vi "Saccade suppression - continuous flash.vi"() -> ()   [LabVIEW 2013]
uses:
  <vilib>/Platform/TimedLoop/XDataNode/timing_clust.ctl
  <vilib>/Platform/TimedLoop/XDataNode/nitl_modes.ctl
  <vilib>/Platform/TimedLoop/XDataNode/wakeup.ctl
  <vilib>/gmath/statdist.llb/Uniform (Discrete) Random.vi
  Eye tracking dependencies/Global 1.vi
  <vilib>/platform/TimedLoop/XDataNode/XDataNode.xnode
  <vilib>/Platform/TimedLoop/XDataNode/XDNodeRunTimeDep.lvlib
  <vilib>/gmath/NI_Gmath.lvlib
panel:
  out "Eye tracker":bool=TRUE
  out "Std name":string="70915_animal15-21_exp1"
  out "Blank":bool
  out "Total number of trials":i32=200
  out "Running!":bool
  in  "Location":string="D:\\Satoru\\Documents\\Attention_Beh_Data\\"
  out "File name exists!":bool
  out "Current trial #":u16
  out "LED":bool
  in  "Abort":bool caption="run-stop"
  in  "File name":string="animal15-29_exp1"
  in  "Save data":bool
  out "State Missed":bool
  out "VS missed":bool
  out "State busy":bool
  out "VS busy":bool
  in  "Tab Control":T1(tab)=enum."Network"
  in  "Notes":string
  in  "Start recording @":string
  in  "Inserted probe @":string
  in  "Brain region":string
  in  "Anesthesia @":string
  in  "Anesthesia":string
  in  "Probe configuration":string
  in  "Probe use number":string
  in  "Probe ID":string
  in  "Probe type":string
  in  "Electrode spacing":string
  in  "Electrode area":string
  in  "Penetration angle (to pia)":string
  in  "Penetration coordinates":string
  in  "Penetration distance":string
  in  "Penetration number":string
  in  "Genotype":string
  in  "Transfection":string
  in  "Mass":string
  in  "Sex":string
  in  "Age":string
  in  "Animal ID":string="14-4"
  in  "inter flash interval (ms)":dbl=300.0
  in  "Max jitter (ms)":dbl=250.0
  in  "VS type":string="continuous_flash"
  in  "Background luminance":sgl
  in  "Pulse amp 0":sgl
  in  "Pulse amp 1":sgl
  in  "Pulse delay (ms)":sgl
  in  "Pulse width (ms)":sgl
  in  "Pulse period":sgl
  in  "Pulse #":sgl
  in  "LED mode":u16(ring) items=["No LED", "Regular", "Random"]
  in  "Chance (%)":dbl
  in  "# of trials":i32=200
  in  "run-stop":bool
  in  "movement":sgl=3.0
  in  "Flash luminance":sgl=100.0
  in  "flash duration (ms)":dbl=48.0
  in  "VS subtype":string="fullfield"
  in  "Include blanks":bool=TRUE
  in  "# of blank trials":i32=200
  in  "Give reward":bool
  in  "Manually give shock":bool
  in  "Water duration (ms)":u32=30
  in  "Shock duration (ms)":u32=10
  in  "Water refractory period (ms)":u32=500
  in  "Shock refractory period (ms)":u32=1000
  in  "Trial timeout (ms)":u32=3000
  in  "Track eye":bool=TRUE
  in  "Allow shock":bool
  in  "Allow timeout":bool
  in  "Manually give water":bool
  in  "Reward period (ms)":u32
  in  "Reward start delay (ms)":u32
  in  "Lick threshold (V)":fxp<+,32,16>=1.600006103515625
  in  "VS threshold (V)":fxp<+,32,16>=0.5
  out "Originating IP":string="192.168.137.2"
  out "Incoming data":string="TrlDone 1.000 "
  in  "Update cycle (ms)":dbl=50.0
  in  "Local IP_This computer":string="192.168.137.10"
  in  "Remote IP_Broadcast":string="192.168.137.255"
  in  "Remote IP_State machine":string="192.168.137.2"
  in  "Remote IP_Visual stimulation":string="192.168.137.3"
  in  "Local port":u16=9090
  in  "Remote port":u16=9091
  out "Error 2":string
  # "Saccade suppression project"
  # "Current trial"
  # "of"
  # "System Status"
  # "VS"
  # "State machine"
  # "Busy"
  # "Missed trial"
  # "Max 20 characters"
  # "(w/o LED)"
  # "Movement threshold (degrees)"
  # "MAX 199.9988"
  # "(This will add trials to the # of trials specified above)"
  # "Errors for debugging"
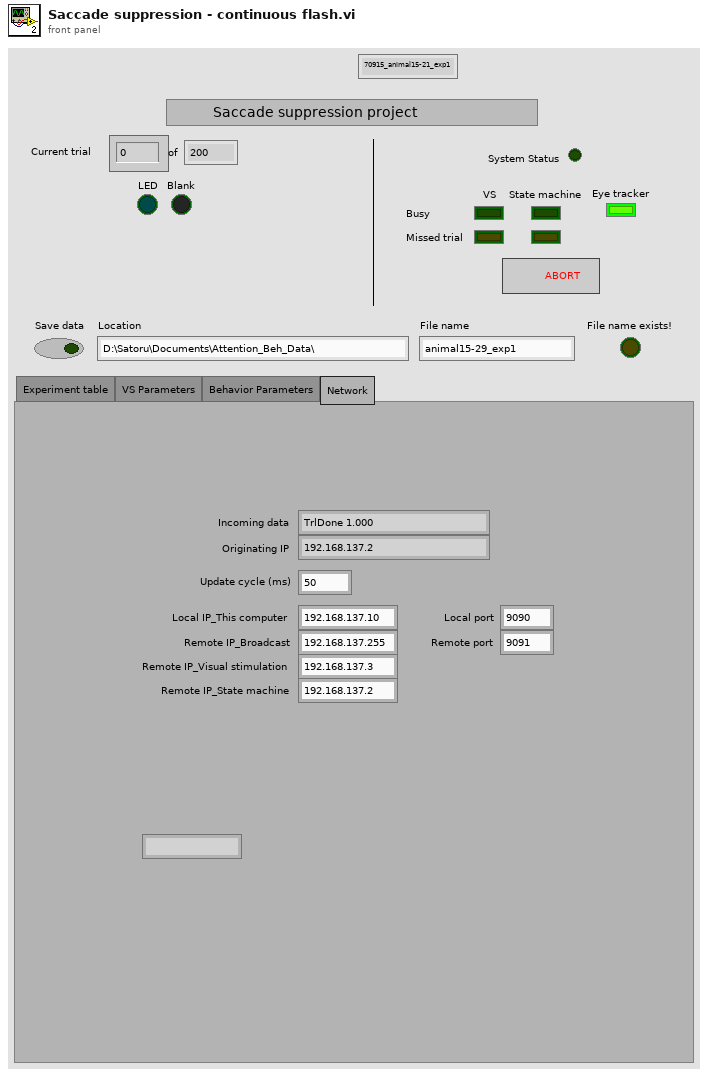
[diagram p1: front panel]
types:
  T1 = enum32{"Experiment table", "VS Parameters", "Behavior Parameters", "Network"}
  T2 = typedef "XDNodeRunTimeDep.lvlib/timing_clust.ctl" = cluster{"Expected End [f-1]":u64, "Actual End [f-1]":u64, "Finished Late? [f-1]":bool, "Expected End [i-1]":u64, "Actual End [i-1]":u64, "Finished Late? [i-1]":bool, "Expected Start [i]":u64, "Actual Start [i]":u64, "Expected Start [f]":u64, "Actual Start [f]":u64, "Source Name":string, "Structure Name":string, "Period":i64, "Deadline":i64, "Offset":i64, "Start":i64, "Priority":i32, "Timeout":i32, "Mode":T3, "Wakeup Reason":T4, "Error":errorcluster, "Source Type":string, "Secondary Source Type":string, "Global End Time":u64, "Global Start Time":u64, "Frame Duration":u64, "Iteration Duration":u64, "Assigned CPU":i32, "I/O Scan Engine Mode":u32}
  T3 = typedef "XDNodeRunTimeDep.lvlib/nitl_modes.ctl" = enum32{"No Change", "Process missed periods, maintain original phase", "Discard missed periods, maintain original phase", "Process missed periods, ignore original phase", "Discard missed periods, ignore original phase"}
  T4 = typedef "XDNodeRunTimeDep.lvlib/wakeup.ctl" = enum32{"Normal", "Aborted", "Asynchronous wakeup", "Timing source error", "Timed loop error", "Timeout"}
  T5 = enum16{"big-endian, network order", "native, host order", "little-endian"}
  T6 = enum16{"open", "replace", "create", "open or create", "replace or create", "replace or create with confirmation"}
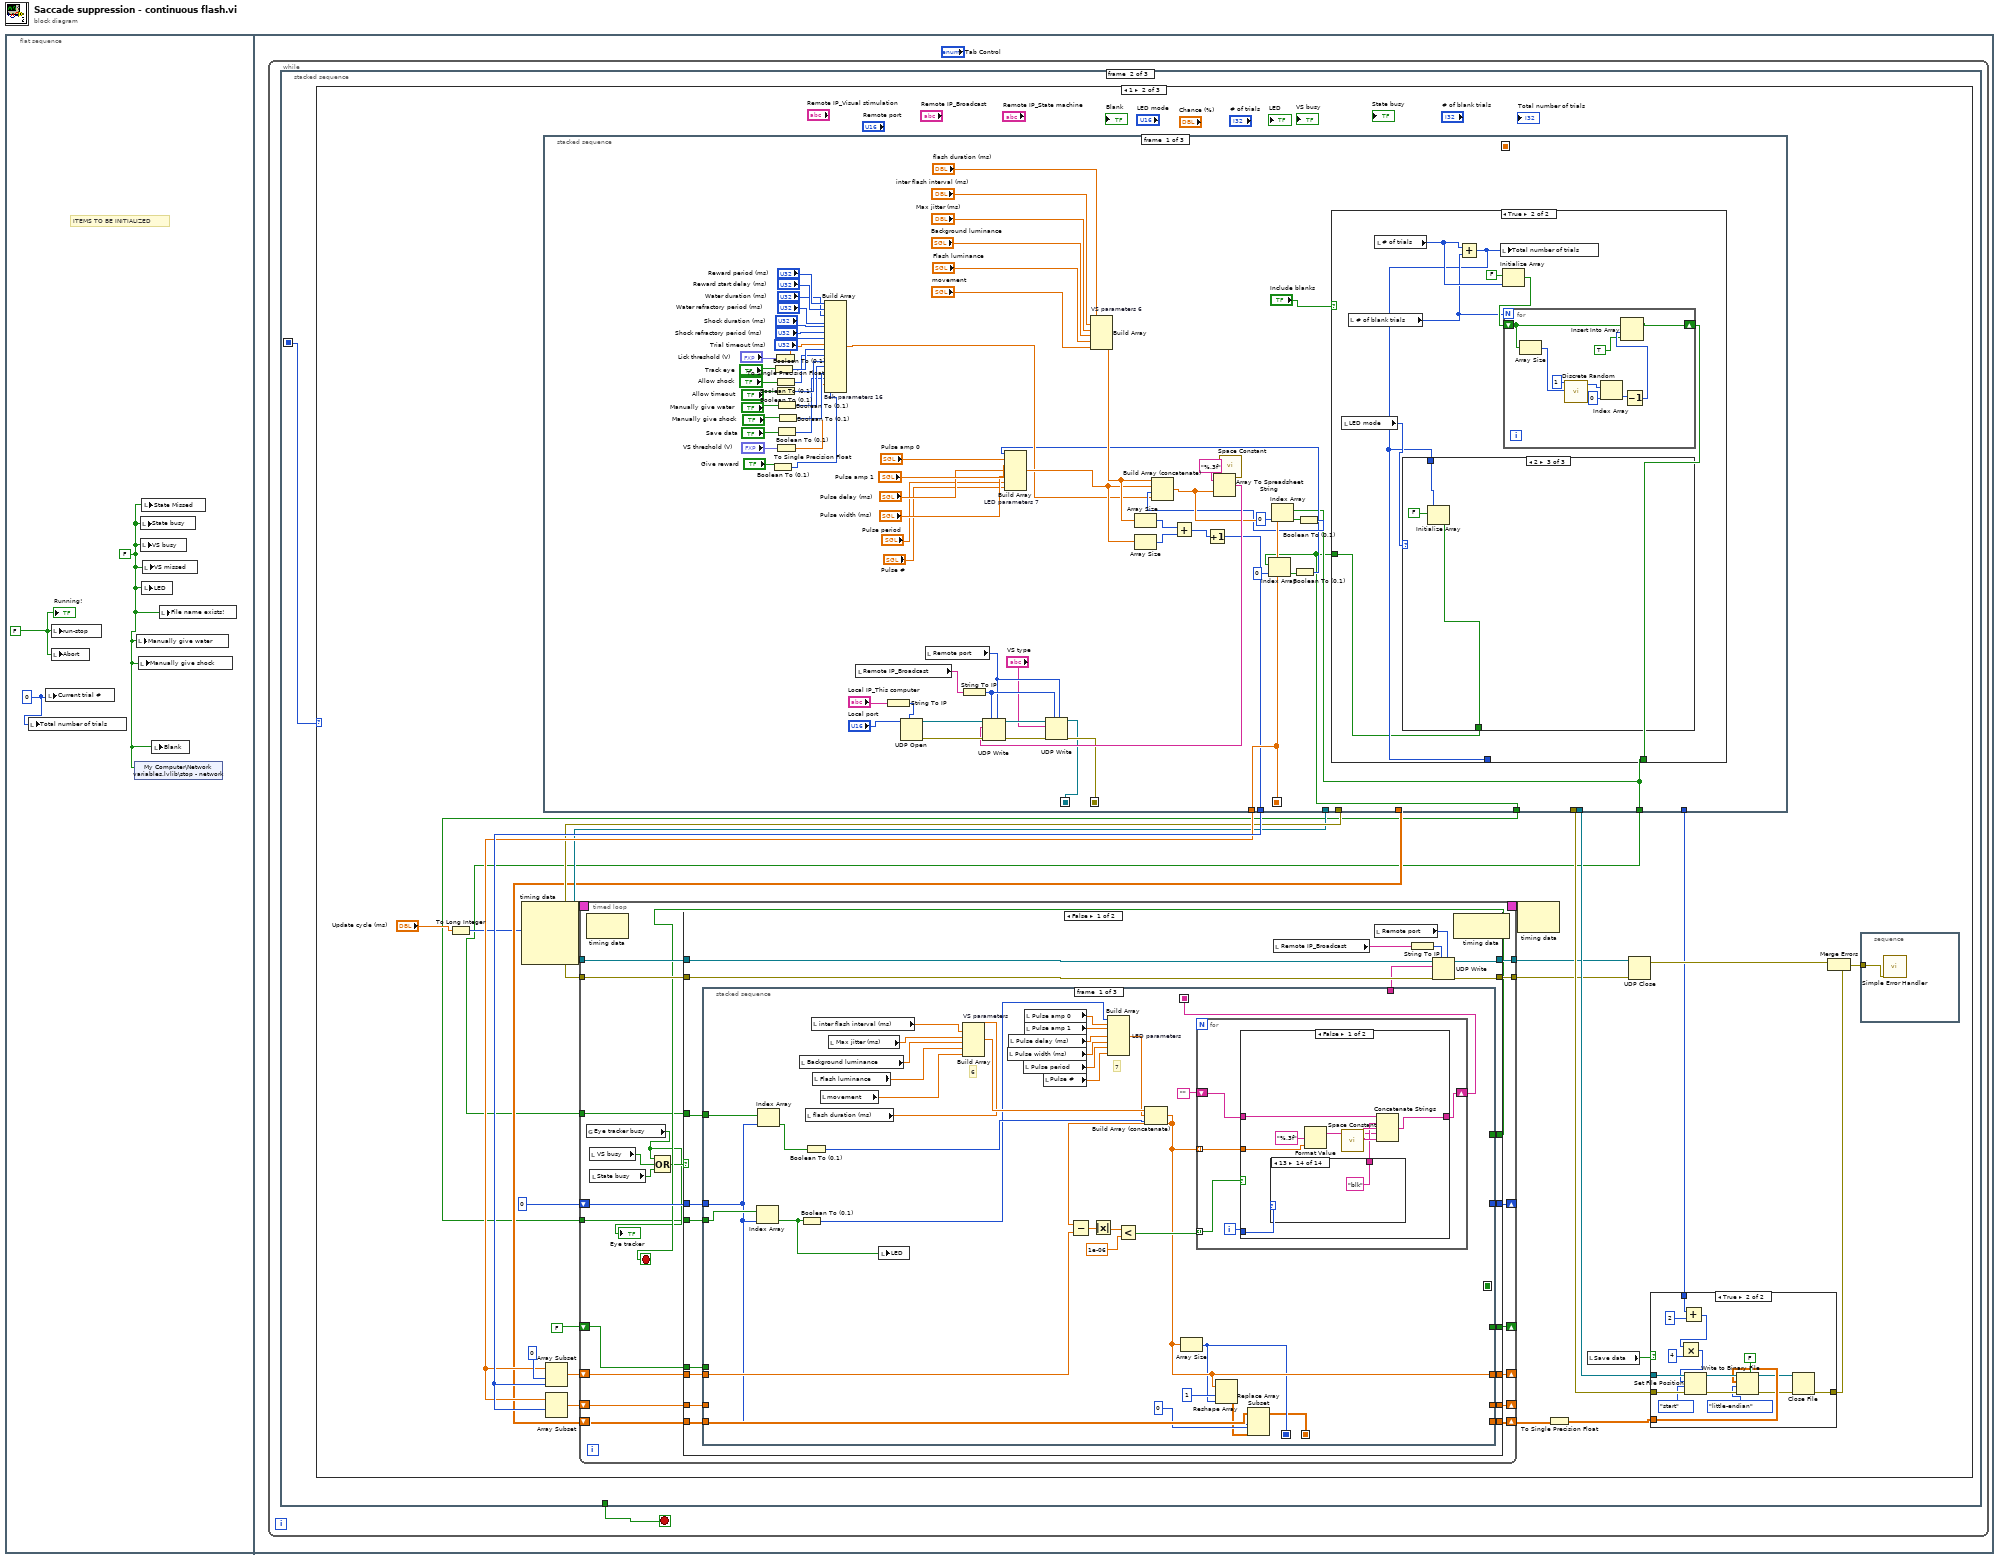
[diagram p0: block diagram]
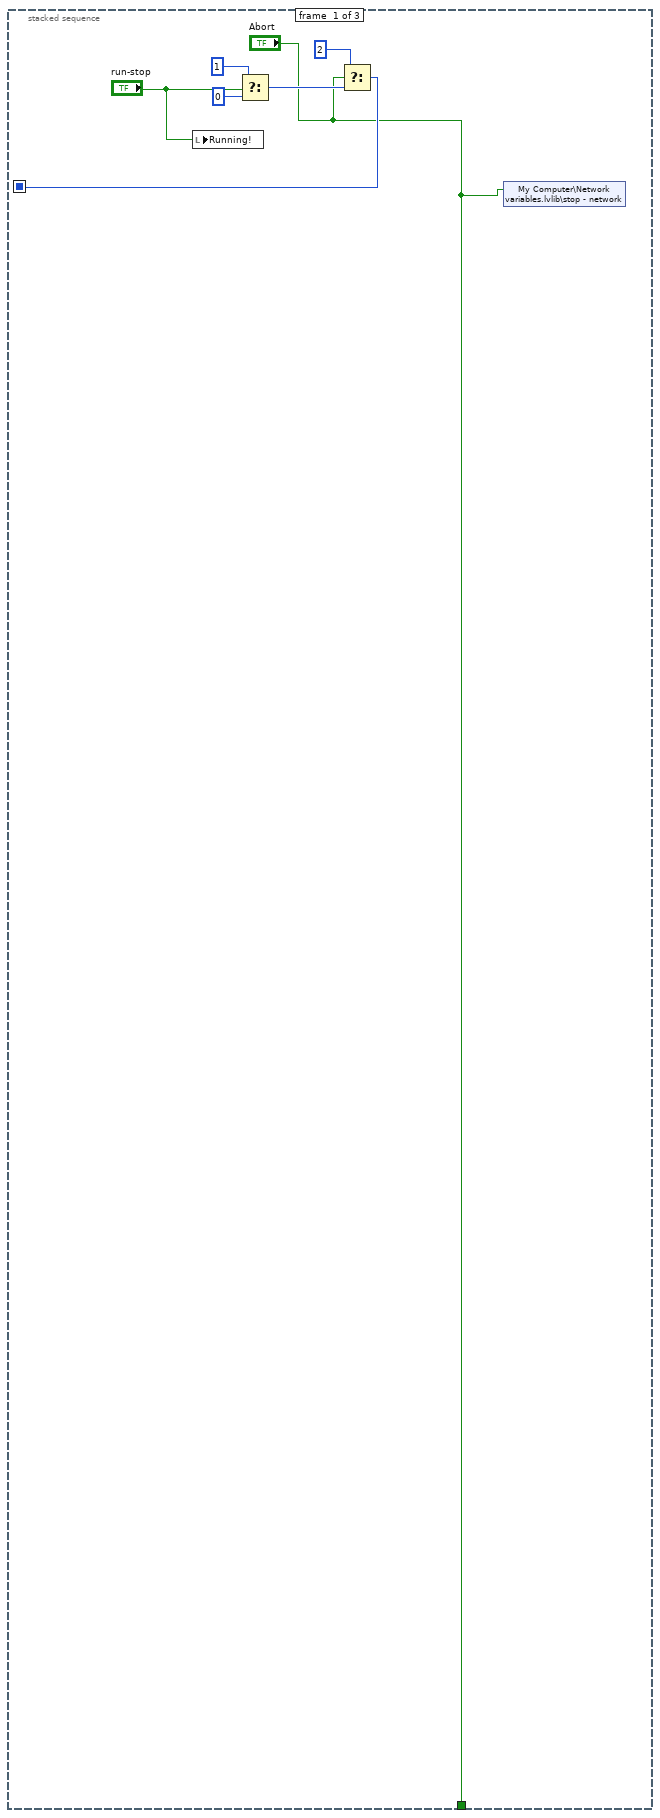
[diagram p2: hidden frame]
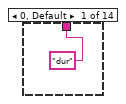
[diagram p4: hidden frame]
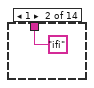
[diagram p5: hidden frame]
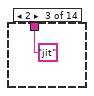
[diagram p6: hidden frame]
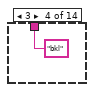
[diagram p7: hidden frame]
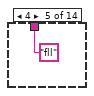
[diagram p8: hidden frame]
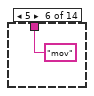
[diagram p9: hidden frame]
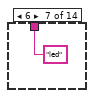
[diagram p10: hidden frame]
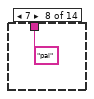
[diagram p11: hidden frame]
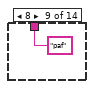
[diagram p12: hidden frame]
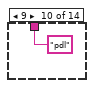
[diagram p13: hidden frame]
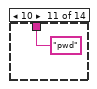
[diagram p14: hidden frame]
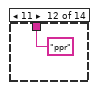
[diagram p15: hidden frame]
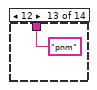
[diagram p16: hidden frame]
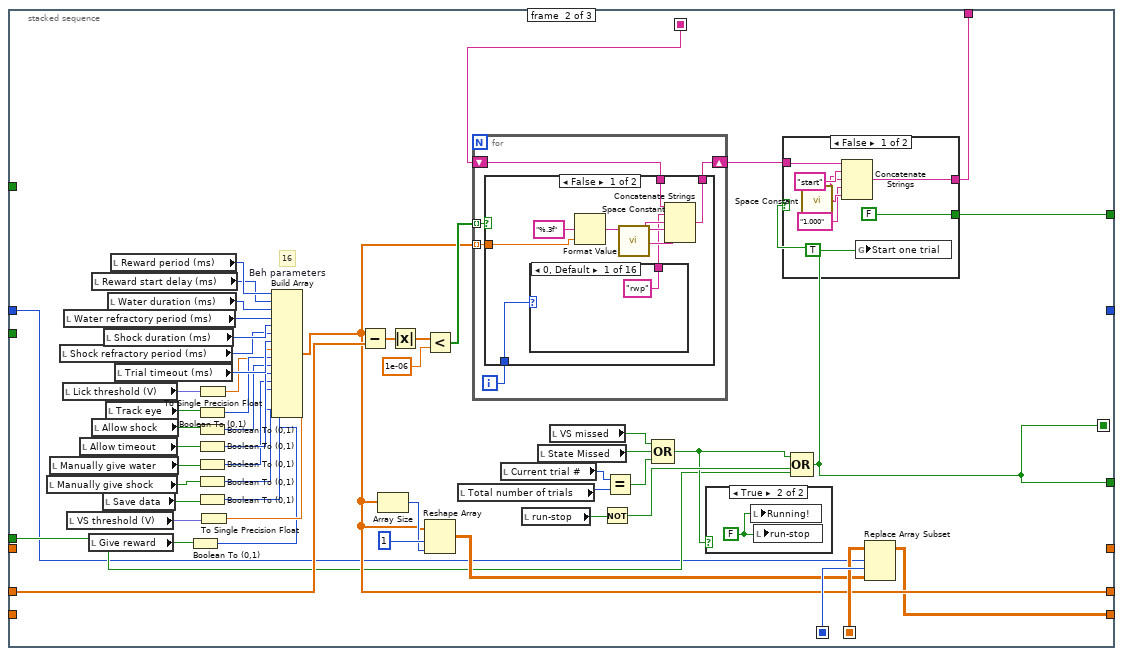
[diagram p18: hidden frame]
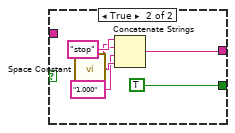
[diagram p20: hidden frame]
diagram:
  n1 = flat-sequence {
    frame #0 {
      w2 = u16 0
      w1 = FALSE ("L dist ind")
      w3 = FALSE
      # "ITEMS TO BE INITIALIZED"
      n2 = local write "Total number of trials"(w2) -> ()
      n3 = local write "Current trial #"(w2) -> ()
      n4 = local write "run-stop"(w3) -> ()
      n5 = local write "Abort"(w3) -> ()
      n6 = shared-variable "My Computer\\Network variables.lvlib\\stop - network"(w1) -> ()  [unwired: 1 in, 1 out]
      n7 = local write "Manually give water"(w1) -> ()
      n8 = local write "Manually give shock"(w1) -> ()
      n9 = local write "State busy"(w1) -> ()
      n10 = local write "VS busy"(w1) -> ()
      n11 = local write "State Missed"(w1) -> ()
      n12 = local write "LED"(w1) -> ()
      n13 = local write "VS missed"(w1) -> ()
      n14 = local write "Blank"(w1) -> ()
      n15 = local write "File name exists!"(w1) -> ()
      "Running!" <- w3
    }
    frame #1 {
      n16 = while {
        stop <- w4 stop-if-true
        n17 = stacked-sequence {
          seq-local: [w7 _ _] -> [_ w12 _]
          tunnel: ["Abort" _ _] -> w4
          frame #0 {
            n18 = local write "Running!"("run-stop") -> ()
            n19 = Select(t=u8 1, s="run-stop", f=u8 0) -> (s? t:f=w8:u8)
            n20 = Select(t=u8 2, s="Abort", f=w8) -> (s? t:f=w7:u8)
            n21 = shared-variable "My Computer\\Network variables.lvlib\\stop - network"("Abort") -> ()  [unwired: 1 in, 1 out]
          }
          frame #1 {
            n22 = case shown="1" w12 {
              frame 0, Default {
              }
              frame 1 {
                n23 = To Long Integer(number="Update cycle (ms)") -> (32bit integer=w22:i32)
                n24 = node-c288(w22) -> (w39:T2)  [unwired: 3 in]
                n25 = stacked-sequence {
                  seq-local: [w439 _ _] -> [_ _ w590]
                  seq-local: [_ w532 _] -> [_ _ w581]
                  seq-local: [w450 _ _] -> [_ _ w579]
                  seq-local: [w449 _ _] -> [_ _ w565]
                  tunnel: [w439 _ _] -> w34
                  tunnel: [w435 _ _] -> w35
                  tunnel: [_ _ w563] -> w31
                  tunnel: [_ _ w562] -> w30
                  tunnel: [_ _ w584] -> w29
                  tunnel: [_ _ w583] -> w25
                  tunnel: [_ _ w582] -> w24
                  tunnel: [_ _ w560] -> w15
                  tunnel: [w431 _ _] -> w14
                  tunnel: [w430 _ _] -> w13
                  frame #0 {
                    n26 = Boolean To (0,1)(Boolean="Give reward") -> (0, 1=w451:i16)
                    n27 = Boolean To (0,1)(Boolean="Track eye") -> (0, 1=w491:i16)
                    n28 = To Single Precision Float(number="Lick threshold (V)") -> (single precision float=w456:sgl)
                    n29 = Boolean To (0,1)(Boolean="Allow shock") -> (0, 1=w489:i16)
                    n30 = Boolean To (0,1)(Boolean="Allow timeout") -> (0, 1=w487:i16)
                    n31 = Boolean To (0,1)(Boolean="Manually give water") -> (0, 1=w485:i16)
                    n32 = Boolean To (0,1)(Boolean="Save data") -> (0, 1=w482:i16)
                    n33 = To Single Precision Float(number="VS threshold (V)") -> (single precision float=w453:sgl)
                    n34 = Boolean To (0,1)(Boolean="Manually give shock") -> (0, 1=w484:i16)
                    n35 = Build Array "Beh parameters 16"("Reward period (ms)", "Reward start delay (ms)", "Water duration (ms)", "Water refractory period (ms)", "Shock duration (ms)", "Shock refractory period (ms)", "Trial timeout (ms)", w456, w491, w489, w487, w485, w484, w482, w453, w451) -> (w437:sgl[])
                    n36 = local read "Remote IP_Broadcast"() -> (w469:string)
                    n37 = String To IP(1:"Local IP_This computer") -> (0:w473:u32)
                    n38 = UDP Open(7:w473, 11:"Local port") -> (port=w470:refnum<k16>, 0:w474:errorcluster)  [unwired: 3 in, 1 out]
                    n39 = local read "Remote port"() -> (w464:u16)
                    n40 = String To IP(1:w469) -> (0:w465:u32)
                    n41 = Build Array "VS parameters 6"("flash duration (ms)", "inter flash interval (ms)", "Max jitter (ms)", "Background luminance", "Flash luminance", "movement") -> (w460:dbl[])
                    n42 = Array Size(array=w460) -> (size(s)=w458:i32)
                    n43 = call <vilib>:"Space Constant.vi"() -> ("String"=w467:string)
                    n44 = case shown="True" "Include blanks" {
                      tunnel: [w503 w510] -> w431
                      tunnel: [w501 w506] -> _
                      tunnel: [w500 w505] -> w430
                      frame False {
                        n45 = local read "# of trials"() -> (w501:i32)
                        n46 = Initialize Array(FALSE, w501) -> (w500:bool[])
                        n47 = Initialize Array(FALSE, w501) -> (w503:bool[])
                        n48 = local write "Total number of trials"(w501) -> ()
                      }
                      frame True {
                        n49 = local read "LED mode"() -> (w507:u16)
                        n50 = local read "# of blank trials"() -> (w508:i32)
                        n51 = local read "# of trials"() -> (w509:i32)
                        n52 = Add(x=w509, y=w508) -> (x+y=w506:i32)
                        n53 = case shown="2" w507 {
                          tunnel: w506 -> [w515 w518 w521]
                          tunnel: [w514 w516 w519] -> w505
                          frame 0, Default {
                            n54 = Initialize Array(FALSE, w515) -> (w514:bool[])
                          }
                          frame 1 {
                            n55 = Initialize Array(FALSE, w518) -> (w516:bool[])
                          }
                          frame 2 {
                            n56 = Initialize Array(FALSE, w521) -> (w519:bool[])
                          }
                        }
                        n57 = local write "Total number of trials"(w506) -> ()
                        n58 = Initialize Array(FALSE, w509) -> (w511:bool[])
                        n59 = for {
                          N: w508 -> [_]
                          shift-right: [w524] -> w510
                          shift-left: w511 -> [w525]
                          n60 = Array Size(array=w525) -> (size(s)=w529:i32)
                          n61 = call-poly <vilib>:"Discrete Random.vi"("n"=w529, "samples"=1) -> ("uniform (discrete) random data"=w528:i32[])  [unwired: 8 in, 1 out]
                          n62 = Index Array(array=w528, index=0) -> (element=w526:i32)
                          n63 = Decrement(x=w526) -> (x-1=w523:i32)
                          n64 = Insert Into Array(array=w525, index=w523, new element=TRUE) -> (w524:bool[])
                        }
                      }
                    }
                    n65 = Index Array(array=w430, index=0) -> (element=w433:bool)
                    n66 = Index Array(array=w431, index=0) -> (element=w440:bool)
                    n67 = Boolean To (0,1)(Boolean=w433) -> (0, 1=w432:i16)
                    n68 = Build Array "LED parameters 7"(w432, "Pulse amp 0", "Pulse amp 1", "Pulse delay (ms)", "Pulse width (ms)", "Pulse period", "Pulse #") -> (w459:sgl[])
                    n69 = Array Size(array=w459) -> (size(s)=w457:i32)
                    n70 = Add(x=w458, y=w457) -> (x+y=w436:i32)
                    n71 = Increment(x=w436) -> (x+1=w435:i32)
                    n72 = Boolean To (0,1)(Boolean=w440) -> (0, 1=w438:i16)
                    n73 = Build Array (concatenate)(w460, w459, w438, w437) -> (w439:dbl[])
                    n74 = Array To Spreadsheet String(delimiter (Tab)=w467, array=w439, 3:"%.3f" ("format string")) -> (spreadsheet string=w466:string)
                    n75 = UDP Write(address=w465, port or service name=w464, connection ID=w470, data in=w466, 8:w474) -> (error out=w463:errorcluster, 3:w462:refnum<k16>)  [unwired: 1 in]
                    n76 = UDP Write(address=w465, port or service name=w464, connection ID=w462, data in="VS type", 8:w463) -> (error out=w450:errorcluster, 3:w449:refnum<k16>)  [unwired: 1 in]
                  }
                  frame #1 {
                    w539 = "&" ("string")
                    # "state definition"
                    n77 = local read "inter flash interval (ms)"() -> (w554:dbl)
                    n78 = local read "Total number of trials"() -> (w531:i32)
                    n79 = local read "Max jitter (ms)"() -> (w553:dbl)
                    n80 = local read "VS subtype"() -> (w558:string)
                    n81 = local read "Chance (%)"() -> (w552:dbl)
                    n82 = local read "LED mode"() -> (w555:u16)
                    n83 = local read "VS type"() -> (w559:string)
                    n84 = String To Byte Array(string=w559) -> (unsigned byte array=w557:u8[])
                    n85 = String To Byte Array(string=w558) -> (unsigned byte array=w556:u8[])
                    n86 = Concatenate Strings("idle", w539, "vs before", w539, "vs", w539, "vs after", w539, "cycle end", w539, "reward", w539, "reward refractory", w539, "punish", w539, "punish refractory", w539, "exit", w539, "timeout", w539) -> (w540:string)
                    n87 = Build Array (concatenate)(w557, w556, w555, w531, w554, w553, w552) -> (w536:dbl[])
                    n88 = String To Byte Array(string=w540) -> (unsigned byte array=w534:u8[])
                    n89 = Initialize Array(sgl 0.0 ("element"), 37 ("dimension size")) -> (w535:sgl[])
                    n90 = Build Array (concatenate)(w536, w535, w534) -> (w533:dbl[])
                    n91 = To Single Precision Float(number=w533) -> (single precision float=w532:sgl[])
                  }
                  frame #2 {
                    # "# of parameters, column"
                    n92 = local read "Save data"() -> (w587:bool)
                    n93 = local read "Remote IP_Broadcast"() -> (w573:string)
                    n94 = local read "Remote port"() -> (w571:u16)
                    n95 = String To IP(1:w573) -> (0:w572:u32)
                    n96 = local read "Total number of trials"() -> (w580:i32)
                    n97 = Array Size(array=w590) -> (size(s)=w588:i32)
                    n98 = Build Array(w580, w588) -> (w586:i32[])
                    n99 = Initialize Array(sgl 0.0, w580, w588) -> (w584:sgl[][])
                    n100 = To Single Precision Float(number=w586) -> (single precision float=w585:sgl[])
                    n101 = case shown="True" w587 {
                      tunnel: w585 -> [_ w663]
                      tunnel: w584 -> [_ w662]
                      tunnel: [_ w661] -> w583
                      tunnel: [_ w660] -> w582
                      tunnel: w581 -> [_ w659]
                      tunnel: ["" w595] -> w567
                      tunnel: [_ w594] -> w560
                      frame False {
                      }
                      frame True {
                        w630 = 20 ("dimension size")
                        w600 = 500 ("dimension size")
                        w602 = T5."little-endian" ("byte order (0:big-endian, network order)")
                        w672 = enum16{"start", "end", "current"}."start" ("from (0:start)")
                        # "param array"
                        # "row and col\nfor param array"
                        # "first 500 singles for common params"
                        # "reserve 500 singles"
                        # "write behhavior params"
                        # "datapath"
                        n102 = while {
                          tunnel: [w703] -> w665
                          tunnel: [w702] -> w664
                          tunnel: [w695] -> w595
                          stop <- w700 continue-if-true
                          (unwired) "0" ("replace string (\"\")")
                          w724 = "/"
                          n103 = Get Date/Time String() -> (date string=w726:string)  [unwired: 3 in, 1 out]
                          n104 = Match Pattern(string=w726, regular expression=w724) -> (before substring=w723:string, after substring=w725:string)  [unwired: 1 in, 2 out]
                          n105 = Decimal String To Number(string=w723) -> (number=w718:i32)  [unwired: 2 in, 1 out]
                          n106 = Match Pattern(string=w725, regular expression=w724) -> (before substring=w722:string, after substring=w712:string)  [unwired: 1 in, 2 out]
                          n107 = Number To Decimal String(number=w718, width (-)=i16 2) -> (decimal integer string=w720:string)
                          n108 = call <vilib>:"Space Constant.vi"() -> ("String"=w719:string)
                          n109 = Decimal String To Number(string=w722) -> (number=w715:i32)  [unwired: 2 in, 1 out]
                          n110 = Search and Replace String(input string=w720, search string=w719) -> (result string=w710:string)  [unwired: 6 in, 3 out]
                          n111 = Number To Decimal String(number=w715, width (-)=i16 2) -> (decimal integer string=w717:string)
                          n112 = String Subset(string=w712, offset (0)=2) -> (substring=w708:string)  [unwired: 1 in]
                          n113 = call <vilib>:"Space Constant.vi"() -> ("String"=w716:string)
                          n114 = Search and Replace String(input string=w717, search string=w716, replace string="0" ("replace string (\"\")")) -> (result string=w709:string)  [unwired: 5 in, 3 out]
                          n115 = Concatenate Strings(w710, w709, w708) -> (w698:string)
                          n116 = Concatenate Strings(w698, "_" ("string"), "File name") -> (w695:string)
                          "Std name" <- w695
                          n117 = Concatenate Strings("Location", w698, "_" ("string"), "File name", ".beh" ("string")) -> (w705:string)
                          n118 = Wait (ms)(milliseconds to wait=u32 100) -> ()  [unwired: 1 out]
                          n119 = String To Path(string=w705) -> (path=w704:path)
                          n120 = call <vilib>:"Check if File or Folder Exists.vi"("path"=w704) -> ("error out"=w702:errorcluster, "file or folder exists?"=w700:bool, "dup path"=w703:path)  [unwired: 8 in]
                          "File name exists!" <- w700
                        }
                        n121 = String To Byte Array(string="Animal ID") -> (unsigned byte array=w622:u8[])
                        n122 = String To Byte Array(string="Genotype") -> (unsigned byte array=w613:u8[])
                        n123 = String To Byte Array(string="Age") -> (unsigned byte array=w614:u8[])
                        n124 = String To Byte Array(string="Sex") -> (unsigned byte array=w615:u8[])
                        n125 = String To Byte Array(string="Mass") -> (unsigned byte array=w616:u8[])
                        n126 = String To Byte Array(string="Transfection") -> (unsigned byte array=w617:u8[])
                        n127 = String To Byte Array(string="Penetration number") -> (unsigned byte array=w619:u8[])
                        n128 = String To Byte Array(string="Penetration distance") -> (unsigned byte array=w621:u8[])
                        n129 = String To Byte Array(string="Penetration coordinates") -> (unsigned byte array=w645:u8[])
                        n130 = String To Byte Array(string="Penetration angle (to pia)") -> (unsigned byte array=w646:u8[])
                        n131 = String To Byte Array(string="Electrode area") -> (unsigned byte array=w647:u8[])
                        n132 = String To Byte Array(string="Electrode spacing") -> (unsigned byte array=w648:u8[])
                        n133 = String To Byte Array(string="Probe type") -> (unsigned byte array=w649:u8[])
                        n134 = String To Byte Array(string="Probe ID") -> (unsigned byte array=w650:u8[])
                        n135 = String To Byte Array(string="Probe use number") -> (unsigned byte array=w651:u8[])
                        n136 = String To Byte Array(string="Probe configuration") -> (unsigned byte array=w652:u8[])
                        n137 = String To Byte Array(string="Anesthesia") -> (unsigned byte array=w653:u8[])
                        n138 = String To Byte Array(string="Anesthesia @") -> (unsigned byte array=w654:u8[])
                        n139 = String To Byte Array(string="Brain region") -> (unsigned byte array=w655:u8[])
                        n140 = String To Byte Array(string="Inserted probe @") -> (unsigned byte array=w656:u8[])
                        n141 = String To Byte Array(string="Start recording @") -> (unsigned byte array=w657:u8[])
                        n142 = String To Byte Array(string="Notes") -> (unsigned byte array=w658:u8[])
                        n143 = Build Array(w622, w613, w614, w615, w616, w617, w619, w621, w645, w646, w647, w648, w649, w650, w651, w652, w653, w654, w655, w656, w657, w658) -> (w625:u8[][])
                        n144 = for {
                          tunnel: w625 -> [w692] mode=indexing
                          tunnel: [w691] -> w623 mode=indexing
                          tunnel: w630 -> [w690]
                          n145 = Initialize Array(u8 0 ("element"), w690) -> (w694:u8[])
                          n146 = Replace Array Subset(array=w694, new element=w692) -> (w691:u8[])  [unwired: 1 in]
                        }
                        n147 = Array Size(array=w625) -> (size(s)=w627:i32[])
                        n148 = Index Array(array=w627, index=0) -> (element=w629:i32)
                        n149 = Open/Create/Replace File(file path (use dialog)=w665, error in=w664, operation (0:open)=T6."create", access (0:read/write)=enum16{"read/write", "read-only", "write-only"}."write-only") -> (refnum out=w686:refnum<file>, error out=w685:errorcluster)  [unwired: 2 in, 1 out]
                        n150 = Multiply(x=w630, y=w629) -> (x*y=w598:i32)
                        n151 = Set File Position(offset (in bytes) (0)=i64 0, refnum=w686, from (0:start)=w672, error in=w685) -> (refnum out=w606:refnum<file>, error out=w604:errorcluster)
                        n152 = To Single Precision Float(number=w623) -> (single precision float=w624:sgl[][])
                        n153 = Initialize Array(sgl 0.0 ("element"), w600) -> (w682:sgl[])
                        n154 = Reshape Array(w624, 1 ("dimension size"), w598) -> (w601:sgl[][])
                        n155 = Write to Binary File(file (use dialog)=w606, data=w601, error in=w604, 5:FALSE ("prepend array or string size? (T)"), 9:w602) -> (refnum out=w605:refnum<file>, error out=w603:errorcluster)  [unwired: 1 in, 1 out]
                        n156 = Write to Binary File(file (use dialog)=w605, data=w682, error in=w603, 5:FALSE ("prepend array or string size? (T)"), 9:w602) -> (refnum out=w680:refnum<file>, error out=w679:errorcluster)  [unwired: 1 in, 1 out]
                        n157 = Multiply(x=w598, y=4) -> (x*y=w599:i32)
                        n158 = Set File Position(offset (in bytes) (0)=w599, refnum=w680, from (0:start)=w672, error in=w679) -> (refnum out=w678:refnum<file>, error out=w677:errorcluster)
                        n159 = Add(x=w598, y=w600) -> (x+y=w594:i32)
                        n160 = Write to Binary File(file (use dialog)=w678, data=w659, error in=w677, 5:FALSE ("prepend array or string size? (T)"), 9:w602) -> (refnum out=w676:refnum<file>, error out=w675:errorcluster)  [unwired: 1 in, 1 out]
                        n161 = Multiply(x=w594, y=4) -> (x*y=w674:i32)
                        n162 = Set File Position(offset (in bytes) (0)=w674, refnum=w676, from (0:start)=w672, error in=w675) -> (refnum out=w670:refnum<file>, error out=w669:errorcluster)
                        n163 = Write to Binary File(file (use dialog)=w670, data=w663, error in=w669, 5:FALSE ("prepend array or string size? (T)"), 9:w602) -> (refnum out=w668:refnum<file>, error out=w667:errorcluster)  [unwired: 1 in, 1 out]
                        n164 = Write to Binary File(file (use dialog)=w668, data=w662, error in=w667, 5:FALSE ("prepend array or string size? (T)"), 9:w602) -> (refnum out=w660:refnum<file>, error out=w661:errorcluster)  [unwired: 1 in, 1 out]
                      }
                    }
                    n165 = String Length(string=w567) -> (length=w570:i32)
                    n166 = Not Equal To 0?(x=w570) -> (x != 0?=w569:bool)
                    n167 = Select(t=w567, s=w569, f="Test") -> (s? t:f=w566:string)
                    n168 = UDP Write(address=w572, port or service name=w571, connection ID=w565, data in=w566, 8:w579) -> (error out=w578:errorcluster, 3:w564:refnum<k16>)  [unwired: 1 in]
                    n169 = UDP Write(address=w572, port or service name=w571, connection ID=w564, data in="VS subtype", 8:w578) -> (error out=w574:errorcluster, 3:w562:refnum<k16>)  [unwired: 1 in]
                    n170 = Unbundle By Name(w574) -> ("code"=w577:i32)
                    n171 = Equal?(x=w577, y=56) -> (x = y?=w575:bool)
                    n172 = case shown="True" w575 {
                      tunnel: w574 -> [w591 _]
                      tunnel: [w591 errorcluster {"status"=FALSE, "code"=0, "source"=""} ("error out")] -> w563
                      frame False {
                      }
                      frame True {
                      }
                    }
                  }
                }
                n173 = Array Subset(array=w34, index=0, length=w35) -> (w37:dbl[])
                n174 = Array Subset(array=w34, index=w35) -> (w33:dbl[])  [unwired: 1 in]
                n175 = timed-loop {
                  shift-right: [w59] -> _
                  shift-left: u16 0 -> [w58]
                  tunnel: w31 -> [w57]
                  tunnel: w30 -> [w56]
                  tunnel: [w55] -> w16
                  tunnel: [w54] -> w17
                  shift-right: [w53] -> _
                  shift-left: w37 -> [w61]
                  shift-right: [w52] -> _
                  shift-left: w33 -> [w60]
                  shift-right: [w50] -> w28
                  shift-left: w29 -> [w51]
                  shift-right: [w49] -> _
                  shift-left: FALSE -> [w48]
                  timing: w39 -> [_]
                  timing-out: [_] -> w38
                  tunnel: w14 -> [w42]
                  tunnel: w13 -> [w41]
                  stop <- w47 stop-if-true
                  n176 = node-c288() -> ()  [unwired: 1 in, 1 out]
                  n177 = global read "Global 1.vi" "Eye tracker busy"() -> (w43:bool)
                  "Eye tracker" <- w43
                  n178 = local read "VS busy"() -> (w45:bool)
                  n179 = local read "State busy"() -> (w44:bool)
                  n180 = Compound Arithmetic op=OR(w43, w45, w44) -> (w46:bool)
                  n181 = case shown="False" w46 {
                    tunnel: w61 -> [w84 w262]
                    tunnel: w60 -> [w83 w260]
                    tunnel: [w82 w251] -> w59
                    tunnel: w58 -> [w81 w252]
                    tunnel: w57 -> [w77 w258]
                    tunnel: w56 -> [w76 w256]
                    tunnel: [w75 w257] -> w55
                    tunnel: [w74 w255] -> w54
                    tunnel: [w73 w262] -> w53
                    tunnel: [w72 w253] -> w52
                    tunnel: w51 -> [w71 w261]
                    tunnel: [w70 w261] -> w50
                    tunnel: [w69 w254] -> w49
                    tunnel: w48 -> [w68 w259]
                    tunnel: [w66 FALSE] -> w47
                    tunnel: w42 -> [w65 _]
                    tunnel: w41 -> [w64 _]
                    frame False {
                      n182 = stacked-sequence {
                        seq-local: [w106 _ _] -> [_ w173 _]
                        seq-local: [w99 _ _] -> [_ w167 _]
                        seq-local: [w98 _ _] -> [_ w166 _]
                        seq-local: [_ w156 _] -> [_ _ w243]
                        tunnel: w81 -> [w87 w154 w245]
                        tunnel: w84 -> [w111 _ _]
                        tunnel: w83 -> [_ w180 _]
                        tunnel: [_ _ w244] -> w82
                        tunnel: [w103 _ _] -> w73
                        tunnel: [_ w163 _] -> w72
                        tunnel: w71 -> [w102 _ _]
                        tunnel: [_ w161 _] -> w70
                        tunnel: [_ w156 _] -> w69
                        tunnel: w68 -> [_ w157 _]
                        tunnel: [_ w155 _] -> w67
                        tunnel: [_ w148 _] -> w66
                        tunnel: w65 -> [w91 _ _]
                        tunnel: w64 -> [w88 _ _]
                        frame #0 {
                          # "6"
                          # "7"
                          n183 = Index Array(array=w88, index=w87) -> (element=w85:bool)
                          n184 = Index Array(array=w91, index=w87) -> (element=w90:bool)
                          n185 = local read "Background luminance"() -> (w95:sgl)
                          n186 = Boolean To (0,1)(Boolean=w85) -> (0, 1=w86:i16)
                          n187 = Boolean To (0,1)(Boolean=w90) -> (0, 1=w89:i16)
                          n188 = local read "flash duration (ms)"() -> (w92:dbl)
                          n189 = local read "inter flash interval (ms)"() -> (w97:dbl)
                          n190 = local read "Flash luminance"() -> (w94:sgl)
                          n191 = local read "movement"() -> (w93:sgl)
                          n192 = local read "Max jitter (ms)"() -> (w96:dbl)
                          n193 = local write "LED"(w85) -> ()
                          n194 = Build Array "VS parameters"(w92, w97, w96, w95, w94, w93) -> (w113:dbl[])
                          n195 = local read "Pulse width (ms)"() -> (w117:sgl)
                          n196 = local read "Pulse delay (ms)"() -> (w116:sgl)
                          n197 = local read "Pulse period"() -> (w118:sgl)
                          n198 = local read "Pulse amp 0"() -> (w114:sgl)
                          n199 = local read "Pulse amp 1"() -> (w115:sgl)
                          n200 = local read "Pulse #"() -> (w119:sgl)
                          n201 = Build Array "LED parameters"(w86, w114, w115, w116, w117, w118, w119) -> (w112:sgl[])
                          n202 = Build Array (concatenate)(w113, w112, w89) -> (w103:dbl[])
                          n203 = Subtract(x=w103, y=w111) -> (x-y=w110:dbl[])
                          n204 = Absolute Value(x=w110) -> (abs(x)=w108:dbl[])
                          n205 = Less?(x=w108, y=1e-06) -> (x < y?=w107:bool[])
                          n206 = Array Size(array=w103) -> (size(s)=w99:i32)
                          n207 = for {
                            tunnel: w107 -> [w124] mode=indexing
                            shift-right: [w122] -> w106
                            shift-left: "" -> [w123]
                            tunnel: w103 -> [w121] mode=indexing
                            i -> [w120]
                            n208 = case shown="False" w124 {
                              tunnel: w123 -> [w132 w147]
                              tunnel: [w131 w147] -> w122
                              tunnel: w120 -> [w129 _]
                              tunnel: w121 -> [w125 _]
                              frame False {
                                n209 = case shown="13" w129 {
                                tunnel: ["dur" "ifi" "jit" "bkl" "fll" "mov" "led" "pai" "paf" "pdl" "pwd" "ppr" "pnm" "blk"] -> w128
                                frame 0, Default {
                                }
                                frame 1 {
                                }
                                frame 2 {
                                }
                                frame 3 {
                                }
                                frame 4 {
                                }
                                frame 5 {
                                }
                                frame 6 {
                                }
                                frame 7 {
                                }
                                frame 8 {
                                }
                                frame 9 {
                                }
                                frame 10 {
                                }
                                frame 11 {
                                }
                                frame 12 {
                                }
                                frame 13 {
                                }
                                }
                                n210 = Format Value(format string="%.3f", value (0)=w125) -> (output string=w126:string)  [unwired: 1 in]
                                n211 = call <vilib>:"Space Constant.vi"() -> ("String"=w130:string)
                                n212 = Concatenate Strings(w132, w128, w130, w126, w130) -> (w131:string)
                              }
                              frame True {
                              }
                            }
                          }
                          n213 = Reshape Array(w103, 1 ("dimension size"), w99) -> (w100:dbl[][])
                          n214 = Replace Array Subset(array=w102, new element=w100, index (row)=w87, index (col)=0) -> (w98:sgl[][])
                        }
                        frame #1 {
                          # "16"
                          n215 = local read "Manually give shock"() -> (w184:bool)
                          n216 = local read "Manually give water"() -> (w186:bool)
                          n217 = local read "Shock refractory period (ms)"() -> (w194:u32)
                          n218 = local read "Lick threshold (V)"() -> (w174:fxp<+,32,16>)
                          n219 = local read "Water refractory period (ms)"() -> (w196:u32)
                          n220 = local read "VS threshold (V)"() -> (w152:fxp<+,32,16>)
                          n221 = local read "Allow timeout"() -> (w188:bool)
                          n222 = local read "Give reward"() -> (w150:bool)
                          n223 = local read "Reward start delay (ms)"() -> (w198:u32)
                          n224 = local read "Allow shock"() -> (w190:bool)
                          n225 = local read "Save data"() -> (w182:bool)
                          n226 = local read "Shock duration (ms)"() -> (w195:u32)
                          n227 = local read "Track eye"() -> (w191:bool)
                          n228 = local read "Water duration (ms)"() -> (w197:u32)
                          n229 = local read "Reward period (ms)"() -> (w199:u32)
                          n230 = local read "Trial timeout (ms)"() -> (w193:u32)
                          n231 = Boolean To (0,1)(Boolean=w150) -> (0, 1=w149:i16)
                          n232 = Boolean To (0,1)(Boolean=w191) -> (0, 1=w192:i16)
                          n233 = Boolean To (0,1)(Boolean=w190) -> (0, 1=w189:i16)
                          n234 = Boolean To (0,1)(Boolean=w188) -> (0, 1=w187:i16)
                          n235 = Boolean To (0,1)(Boolean=w186) -> (0, 1=w185:i16)
                          n236 = Boolean To (0,1)(Boolean=w184) -> (0, 1=w183:i16)
                          n237 = Boolean To (0,1)(Boolean=w182) -> (0, 1=w181:i16)
                          n238 = To Single Precision Float(number=w174) -> (single precision float=w175:sgl)
                          n239 = To Single Precision Float(number=w152) -> (single precision float=w151:sgl)
                          n240 = Build Array "Beh parameters"(w199, w198, w197, w196, w195, w194, w193, w175, w192, w189, w187, w185, w183, w181, w151, w149) -> (w163:sgl[])
                          n241 = Subtract(x=w163, y=w180) -> (x-y=w179:dbl[])
                          n242 = Array Size(array=w163) -> (size(s)=w164:i32)
                          n243 = Absolute Value(x=w179) -> (abs(x)=w177:dbl[])
                          n244 = Less?(x=w177, y=1e-06) -> (x < y?=w176:bool[])
                          n245 = Reshape Array(w163, 1 ("dimension size"), w164) -> (w162:sgl[][])
                          n246 = local read "Total number of trials"() -> (w153:i32)
                          n247 = for {
                            tunnel: w176 -> [w216] mode=indexing
                            tunnel: w163 -> [w215] mode=indexing
                            shift-right: [w213] -> w172
                            shift-left: w173 -> [w214]
                            i -> [w217]
                            n248 = case shown="False" w216 {
                              tunnel: w217 -> [w225 _]
                              tunnel: w215 -> [w223 _]
                              tunnel: w214 -> [w220 w242]
                              tunnel: [w218 w242] -> w213
                              frame False {
                                n249 = case shown="0, Default" w225 {
                                tunnel: ["rwp" "rwd" "wdr" "wre" "shd" "shr" "tto" "lkt" "etk" "ash" "ato" "gwt" "gsh" "sav" "vsh" "rew"] -> w219
                                frame 0, Default {
                                }
                                frame 1 {
                                }
                                frame 2 {
                                }
                                frame 3 {
                                }
                                frame 4 {
                                }
                                frame 5 {
                                }
                                frame 6 {
                                }
                                frame 7 {
                                }
                                frame 8 {
                                }
                                frame 9 {
                                }
                                frame 10 {
                                }
                                frame 11 {
                                }
                                frame 12 {
                                }
                                frame 13 {
                                }
                                frame 14 {
                                }
                                frame 15 {
                                }
                                }
                                n250 = Format Value(format string="%.3f", value (0)=w223) -> (output string=w221:string)  [unwired: 1 in]
                                n251 = call <vilib>:"Space Constant.vi"() -> ("String"=w222:string)
                                n252 = Concatenate Strings(w220, w219, w222, w221, w222) -> (w218:string)
                              }
                              frame True {
                              }
                            }
                          }
                          n253 = local read "Current trial #"() -> (w168:u16)
                          n254 = local read "run-stop"() -> (w160:bool)
                          n255 = local read "State Missed"() -> (w170:bool)
                          n256 = local read "VS missed"() -> (w169:bool)
                          n257 = Not(x=w160) -> (.not. x?=w159:bool)
                          n258 = Equal?(x=w168, y=w153) -> (x = y?=w171:bool)
                          n259 = Compound Arithmetic op=OR(w169, w170, w171) -> (w158:bool)
                          n260 = case shown="True" w158 {
                            frame False {
                            }
                            frame True {
                              w200 = FALSE
                              n261 = local write "Running!"(w200) -> ()
                              n262 = local write "run-stop"(w200) -> ()
                            }
                          }
                          n263 = Compound Arithmetic op=OR(w158, w159, w157) -> (w156:bool)
                          n264 = case shown="False" w156 {
                            tunnel: w172 -> [w207 _]
                            tunnel: [w203 w209] -> w155
                            tunnel: [FALSE TRUE] -> w148
                            frame False {
                              n265 = call <vilib>:"Space Constant.vi"() -> ("String"=w205:string)
                              n266 = Concatenate Strings(w207, "start", w205, "1.000", w205) -> (w203:string)
                              n267 = global write "Global 1.vi" "Start one trial"(TRUE) -> ()
                            }
                            frame True {
                              n268 = call <vilib>:"Space Constant.vi"() -> ("String"=w211:string)
                              n269 = Concatenate Strings("stop", w211, "1.000", w211) -> (w209:string)
                            }
                          }
                          n270 = Replace Array Subset(array=w166, new element=w162, index (row)=w154, index (col)=w167) -> (w161:sgl[][])
                        }
                        frame #2 {
                          n271 = case shown="False" w243 {
                            tunnel: w245 -> [w248 w249]
                            tunnel: [w247 w249] -> w244
                            frame False {
                              w246 = TRUE
                              n272 = Increment(x=w248) -> (x+1=w247:u16)
                              "Current trial #" <- w247
                              n273 = local write "VS busy"(w246) -> ()
                              n274 = local write "State busy"(w246) -> ()
                            }
                            frame True {
                            }
                          }
                        }
                      }
                      n275 = local read "Remote IP_Broadcast"() -> (w78:string)
                      n276 = local read "Remote port"() -> (w80:u16)
                      n277 = String To IP(1:w78) -> (0:w79:u32)
                      n278 = UDP Write(address=w79, port or service name=w80, connection ID=w76, data in=w67, 8:w77) -> (error out=w75:errorcluster, 3:w74:refnum<k16>)  [unwired: 1 in]
                    }
                    frame True {
                      n279 = stacked-sequence {
                        seq-local: [w270 _] -> [_ w366]
                        seq-local: [w269 _] -> [_ w367]
                        tunnel: w260 -> [w286 _]
                        tunnel: w259 -> [w277 _]
                        tunnel: w258 -> [w276 _]
                        tunnel: [_ w361] -> w257
                        tunnel: w256 -> [w275 _]
                        tunnel: [_ w358] -> w255
                        tunnel: [w263 _] -> w254
                        tunnel: [w271 _] -> w253
                        tunnel: w252 -> [_ w355]
                        tunnel: [_ w353] -> w251
                        frame #0 {
                          n280 = local read "Manually give shock"() -> (w296:bool)
                          n281 = local read "Manually give water"() -> (w298:bool)
                          n282 = local read "Shock refractory period (ms)"() -> (w306:u32)
                          n283 = local read "Lick threshold (V)"() -> (w287:fxp<+,32,16>)
                          n284 = local read "Water refractory period (ms)"() -> (w308:u32)
                          n285 = local read "VS threshold (V)"() -> (w267:fxp<+,32,16>)
                          n286 = local read "Allow timeout"() -> (w300:bool)
                          n287 = local read "Reward start delay (ms)"() -> (w310:u32)
                          n288 = local read "Allow shock"() -> (w302:bool)
                          n289 = local read "Save data"() -> (w294:bool)
                          n290 = local read "Shock duration (ms)"() -> (w307:u32)
                          n291 = local read "Track eye"() -> (w303:bool)
                          n292 = local read "Water duration (ms)"() -> (w309:u32)
                          n293 = local read "Reward period (ms)"() -> (w311:u32)
                          n294 = local read "Trial timeout (ms)"() -> (w305:u32)
                          n295 = Boolean To (0,1)(Boolean=w303) -> (0, 1=w304:i16)
                          n296 = Boolean To (0,1)(Boolean=w302) -> (0, 1=w301:i16)
                          n297 = Boolean To (0,1)(Boolean=w300) -> (0, 1=w299:i16)
                          n298 = Boolean To (0,1)(Boolean=w298) -> (0, 1=w297:i16)
                          n299 = Boolean To (0,1)(Boolean=w296) -> (0, 1=w295:i16)
                          n300 = Boolean To (0,1)(Boolean=w294) -> (0, 1=w293:i16)
                          n301 = To Single Precision Float(number=w287) -> (single precision float=w288:sgl)
                          n302 = To Single Precision Float(number=w267) -> (single precision float=w266:sgl)
                          n303 = local read "Give reward"() -> (w265:bool)
                          n304 = Boolean To (0,1)(Boolean=w265) -> (0, 1=w264:i16)
                          n305 = Build Array "Beh parameters"(w311, w310, w309, w308, w307, w306, w305, w288, w304, w301, w299, w297, w295, w293, w266, w264) -> (w271:sgl[])
                          n306 = Subtract(x=w271, y=w286) -> (x-y=w292:dbl[])
                          n307 = Absolute Value(x=w292) -> (abs(x)=w290:dbl[])
                          n308 = Less?(x=w290, y=1e-06) -> (x < y?=w289:bool[])
                          n309 = for {
                            tunnel: w289 -> [w326] mode=indexing
                            tunnel: w271 -> [w325] mode=indexing
                            shift-right: [w323] -> w272
                            shift-left: "" -> [w324]
                            i -> [w327]
                            n310 = case shown="False" w326 {
                              tunnel: w327 -> [w335 _]
                              tunnel: w325 -> [w333 _]
                              tunnel: w324 -> [w330 w352]
                              tunnel: [w328 w352] -> w323
                              frame False {
                                n311 = case shown="0, Default" w335 {
                                tunnel: ["rwp" "rwd" "wdr" "wre" "shd" "shr" "tto" "lkt" "etk" "ash" "ato" "gwt" "gsh" "sav" "vst" "rew"] -> w329
                                frame 0, Default {
                                }
                                frame 1 {
                                }
                                frame 2 {
                                }
                                frame 3 {
                                }
                                frame 4 {
                                }
                                frame 5 {
                                }
                                frame 6 {
                                }
                                frame 7 {
                                }
                                frame 8 {
                                }
                                frame 9 {
                                }
                                frame 10 {
                                }
                                frame 11 {
                                }
                                frame 12 {
                                }
                                frame 13 {
                                }
                                frame 14 {
                                }
                                frame 15 {
                                }
                                }
                                n312 = Format Value(format string="%.3f", value (0)=w333) -> (output string=w331:string)  [unwired: 1 in]
                                n313 = call <vilib>:"Space Constant.vi"() -> ("String"=w332:string)
                                n314 = Concatenate Strings(w330, w329, w332, w331, w332) -> (w328:string)
                              }
                              frame True {
                              }
                            }
                          }
                          n315 = String Length(string=w272) -> (length=w273:i32)
                          n316 = Not Equal To 0?(x=w273) -> (x != 0?=w274:bool)
                          n317 = case shown="True" w274 {
                            tunnel: w276 -> [w312 w318]
                            tunnel: [w312 w317] -> w269
                            tunnel: w275 -> [w313 w316]
                            tunnel: [w313 w315] -> w270
                            tunnel: w272 -> [_ w314]
                            frame False {
                            }
                            frame True {
                              n318 = local read "Remote IP_Broadcast"() -> (w319:string)
                              n319 = local read "Remote port"() -> (w321:u16)
                              n320 = String To IP(1:w319) -> (0:w320:u32)
                              n321 = UDP Write(address=w320, port or service name=w321, connection ID=w316, data in=w314, 8:w318) -> (error out=w317:errorcluster, 3:w315:refnum<k16>)  [unwired: 1 in]
                            }
                          }
                          n322 = local read "Total number of trials"() -> (w268:i32)
                          n323 = local read "Current trial #"() -> (w281:u16)
                          n324 = local read "run-stop"() -> (w280:bool)
                          n325 = local read "State Missed"() -> (w283:bool)
                          n326 = local read "VS missed"() -> (w282:bool)
                          n327 = Not(x=w280) -> (.not. x?=w279:bool)
                          n328 = Equal?(x=w281, y=w268) -> (x = y?=w284:bool)
                          n329 = Compound Arithmetic op=OR(w282, w283, w284) -> (w278:bool)
                          n330 = Compound Arithmetic op=OR(w278, w279, w277) -> (w263:bool)
                          n331 = case shown="True" w263 {
                            frame False {
                            }
                            frame True {
                              w322 = FALSE
                              n332 = local write "Running!"(w322) -> ()
                              n333 = local write "run-stop"(w322) -> ()
                            }
                          }
                        }
                        frame #1 {
                          n334 = UDP Read(connection ID=w366, timeout ms (25000)=0, 8:w367) -> (data out=w354:string, error out=w362:errorcluster, 3:w358:refnum<k16>, 6:w356:u32)  [unwired: 1 in, 1 out]
                          n335 = Unbundle By Name(w362) -> ("code"=w363:i32)
                          n336 = Equal?(x=w363, y=56) -> (x = y?=w365:bool)
                          n337 = case shown="True" w365 {
                            tunnel: w362 -> [w407 _]
                            tunnel: [w407 errorcluster {"status"=FALSE, "code"=0, "source"=""} ("error out")] -> w361
                            frame False {
                            }
                            frame True {
                            }
                          }
                          n338 = String Length(string=w354) -> (length=w360:i32)
                          n339 = Not Equal To 0?(x=w360) -> (x != 0?=w359:bool)
                          n340 = case shown="True" w359 {
                            tunnel: w356 -> [_ w372]
                            tunnel: w355 -> [w368 w371]
                            tunnel: w354 -> [_ w376]
                            tunnel: [w368 w369] -> w353
                            frame False {
                            }
                            frame True {
                              (unwired) -1.0 ("default value 2")
                              (unwired) "no" ("default value 1")
                              n341 = Scan From String(format string="%s %f ", input string=w376, initial scan location=u32 0) -> (output 1=w373:string, output 2=w370:dbl)  [unwired: 3 in, 3 out]
                              n342 = case shown="\"TrlDone\", Default" w373 {
                                tunnel: w372 -> [w384]
                                tunnel: w371 -> [w377]
                                tunnel: w370 -> [w379]
                                tunnel: [w377] -> w369
                                frame "TrlDone", Default {
                                n343 = local read "Remote IP_State machine"() -> (w381:string)
                                n344 = IP To String(1:TRUE ("dot notation? (F)"), 2:w384) -> (0:w378:string)
                                "Originating IP" <- w378
                                n345 = Match True/False String(2:"" ("false string"), 3:w381, 4:w378) -> (0:w380:bool)  [unwired: 1 out]
                                n346 = case shown="False" w380 {
                                tunnel: w377 -> [w385 w404]
                                tunnel: w379 -> [w386 w405]
                                tunnel: w378 -> [w390 _]
                                frame False {
                                n347 = local read "Remote IP_Visual stimulation"() -> (w388:string)
                                n348 = Match True/False String(2:"" ("false string"), 3:w388, 4:w390) -> (0:w387:bool)  [unwired: 1 out]
                                n349 = case shown="True" w387 {
                                tunnel: w386 -> [_ w395]
                                tunnel: w385 -> [_ w394]
                                frame False {
                                "Error 2" <- "Unknown source Error"
                                }
                                frame True {
                                n350 = Subtract(x=w395, y=w394) -> (x-y=w398:dbl)
                                n351 = global write "Global 1.vi" "camera stop"(TRUE ("dot notation? (F)")) -> ()
                                n352 = Absolute Value(x=w398) -> (abs(x)=w397:dbl)
                                n353 = local write "VS busy"(FALSE) -> ()
                                n354 = Greater?(x=w397, y=1e-06) -> (0:→"VS missed":bool)
                                }
                                }
                                }
                                frame True {
                                n355 = Subtract(x=w405, y=w404) -> (x-y=w403:dbl)
                                n356 = local write "State busy"(FALSE) -> ()
                                n357 = Absolute Value(x=w403) -> (abs(x)=w402:dbl)
                                n358 = Greater?(x=w402, y=1e-06) -> (0:→"State Missed":bool)
                                }
                                }
                                }
                              }
                              "Incoming data" <- w376
                            }
                          }
                        }
                      }
                    }
                  }
                  n359 = node-c288() -> ()  [unwired: 1 in, 1 out]
                }
                n360 = node-c288(w38) -> ()  [unwired: 1 out]
                n361 = To Single Precision Float(number=w28) -> (single precision float=w23:sgl[][])
                n362 = local read "Save data"() -> (w26:bool)
                n363 = UDP Close(connection ID=w17, 8:w16) -> (error out=w21:errorcluster)  [unwired: 1 out]
                n364 = case shown="True" w26 {
                  tunnel: w25 -> [w413 w429]
                  tunnel: w24 -> [_ w428]
                  tunnel: w23 -> [_ w420]
                  tunnel: [w413 w417] -> w20
                  tunnel: w15 -> [_ w416]
                  frame False {
                  }
                  frame True {
                    n365 = Add(x=w416, y=2) -> (x+y=w414:i32)
                    n366 = Multiply(x=w414, y=4) -> (x*y=w425:i32)
                    n367 = Set File Position(offset (in bytes) (0)=w425, refnum=w428, from (0:start)=enum16{"start", "end", "current"}."start", error in=w429) -> (refnum out=w422:refnum<file>, error out=w423:errorcluster)
                    n368 = Write to Binary File(file (use dialog)=w422, data=w420, error in=w423, 5:FALSE ("prepend array or string size? (T)"), 9:T5."little-endian" ("byte order (0:big-endian, network order)")) -> (refnum out=w418:refnum<file>, error out=w419:errorcluster)  [unwired: 1 in, 1 out]
                    n369 = Close File(refnum=w418, error in=w419) -> (error out=w417:errorcluster)  [unwired: 1 out]
                  }
                }
                n370 = Merge Errors(w21, w20) -> (w19:errorcluster)
                n371 = stacked-sequence {
                  tunnel: w19 -> [w40]
                  frame #0 {
                    n372 = call <vilib>:"Simple Error Handler.vi"("error in (no error)"=w40) -> ()  [unwired: 4 in, 5 out]
                  }
                }
              }
              frame 2 {
              }
            }
          }
          frame #2 {
            n373 = Wait (ms)(milliseconds to wait=u32 100) -> ()  [unwired: 1 out]
          }
        }
      }
    }
  }
